vi "例9.7 利用声卡连续输出波形.vi"() -> ()   [LabVIEW 2012]
doc: "本VI说明了生成并播放正弦波、方波、锯齿波和三角波的方式。在连续播放时可更改生成波形的频率和类型。"
uses:
  <vilib>/sound2/lvsound2.llb/Sound Data Format.ctl
  <vilib>/sound2/lvsound2.llb/Sampling Mode.ctl
  <vilib>/sound2/lvsound2.llb/Sound Output Set Volume (Single).vi
  <vilib>/sound2/lvsound2.llb/Sound Output Write (DBL).vi
  <vilib>/measure/NI_MABase.lvlib
panel:
  in  "声音格式":T1={"sample rate (S/s)"=44100.0, "number of channels"=2, "bits per sample"=16}
  in  "音量大小":dbl(slide)=70.40816326530613 caption="音量" scale=0.0..100.0
  out "仿真波形":waveform(dbl)[](graph) caption="生成声音"
  in  "频率":dbl=500.0 format="%0.2p"
  in  "stop":bool caption="停止"
  in  "Number of Samples/ch":i32=5000 caption="每通道采样数"
  in  "设备ID":u32
  # "配置"
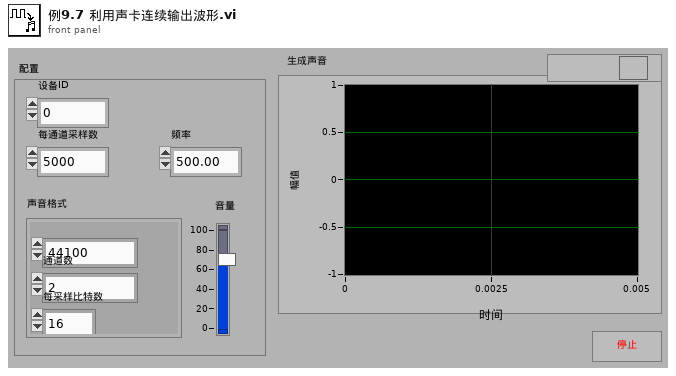
[diagram p1: front panel]
types:
  T1 = typedef "Sound Data Format.ctl" = cluster{"sample rate (S/s)":dbl, "number of channels":i32, "bits per sample":i32}
  T2 = typedef "Sampling Mode.ctl" = i32
  T3 = typedef "Sound Output Task ID.ctl" = u32
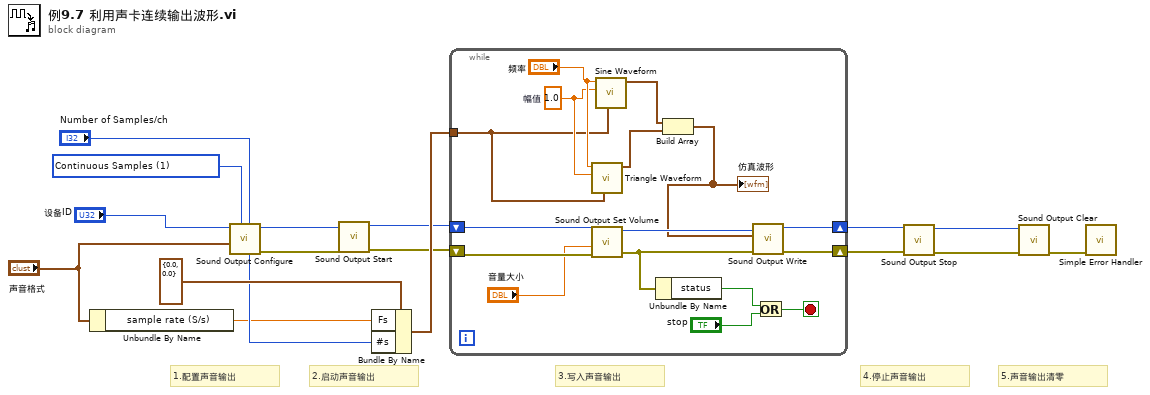
[diagram p0: block diagram]
diagram:
  w16 = T2 1 items=["Finite Samples", "Continuous Samples"] ("sample mode")
  # "4.停止声音输出"
  # "2.启动声音输出"
  # "3.写入声音输出"
  # "5.声音输出清零"
  # "1.配置声音输出"
  n1 = Unbundle By Name("声音格式") -> ("sample rate (S/s)"=w11:dbl)
  n2 = call <vilib>:"Sound Output Configure.vi"("number of samples/ch"="Number of Samples/ch", "sample mode"=w16, "sound format"="声音格式", "device ID"="设备ID") -> ("error out"=w6:errorcluster, "task ID"=w8:T3)  [unwired: 6 in]
  n3 = call <vilib>:"Sound Output Start.vi"("error in (no error)"=w6, "task ID"=w8) -> ("error out"=w5:errorcluster, "task ID out"=w7:T3)  [unwired: 8 in]
  n4 = Bundle By Name(cluster=cluster{"Fs":dbl, "#s":dbl} {"Fs"=0.0, "#s"=0.0} ("sampling info"), "Fs"=w11, "#s"="Number of Samples/ch") -> (w13:cluster{"Fs":dbl, "#s":dbl})
  n5 = while {
    shift-right: [w31] -> w2
    shift-left: w5 -> [w26]
    shift-right: [w32] -> w4
    shift-left: w7 -> [w24]
    tunnel: w13 -> [w20]
    stop <- w29 stop-if-true
    w21 = 1.0  # 幅值
    n6 = call <vilib>:"Triangle Waveform.vi"("sampling info"=w20, "amplitude"=w21, "frequency"="频率") -> ("signal out"=w18:waveform(dbl))  [unwired: 7 in, 1 out]
    n7 = call-poly <vilib>:"Sound Output Set Volume.vi"("error in (no error)"=w26, "volume"="音量大小", "task ID"=w24) -> ("error out"=w27:errorcluster, "task ID out"=w25:T3)  [unwired: 7 in]
    n8 = call <vilib>:"Sine Waveform.vi"("sampling info"=w20, "amplitude"=w21, "frequency"="频率") -> ("signal out"=w19:waveform(dbl))  [unwired: 7 in, 1 out]
    n9 = Unbundle By Name(w27) -> ("status"=w28:bool)
    n10 = Build Array(w19, w18) -> (w17:waveform(dbl)[])
    "仿真波形" <- w17
    n11 = call-poly <vilib>:"Sound Output Write.vi"("error in (no error)"=w27, "data"=w17, "task ID"=w25) -> ("error out"=w31:errorcluster, "task ID out"=w32:T3)  [unwired: 7 in]
    n12 = Or(x=w28, y="stop") -> (x .or. y?=w29:bool)
  }
  n13 = call <vilib>:"Sound Output Stop.vi"("error in (no error)"=w2, "task ID"=w4) -> ("error out"=w1:errorcluster, "task ID out"=w3:T3)  [unwired: 8 in]
  n14 = call <vilib>:"Sound Output Clear.vi"("error in (no error)"=w1, "task ID"=w3) -> ("error out"=w12:errorcluster)  [unwired: 9 in]
  n15 = call <vilib>:"Simple Error Handler.vi"("error in (no error)"=w12) -> ()  [unwired: 4 in, 5 out]
